vi "2-5.vi"() -> ()   [LabVIEW 2022 SP3]
panel:
  out "高压报警警示灯":bool
  out "正常运行指示灯":bool
  out "当前电压值":dbl
  out "当前电压报警上限值":dbl
  in  "确定按钮":bool
  in  "电压报警上限值":dbl
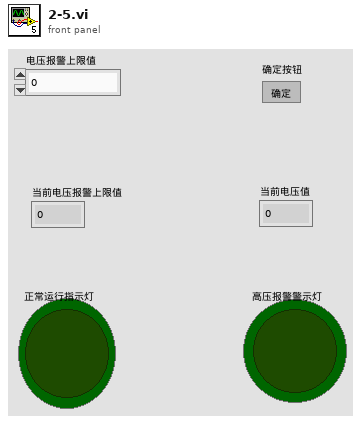
[diagram p1: front panel]
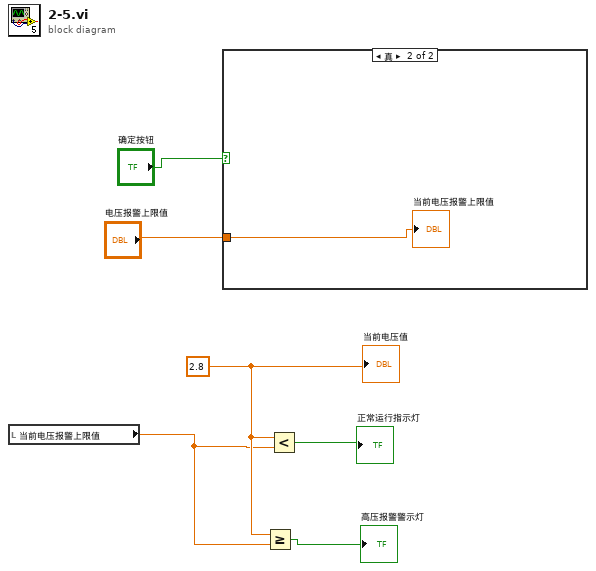
[diagram p0: block diagram]
diagram:
  w2 = 2.8
  n1 = local read "当前电压报警上限值"() -> (w1:dbl)
  n2 = case shown="真" "确定按钮" {
    tunnel: "电压报警上限值" -> [_ w7]
    frame False {
    }
    frame True {
      "当前电压报警上限值" <- w7
    }
  }
  n3 = Greater Or Equal?(x=w2, y=w1) -> (x >= y?=→"高压报警警示灯":bool)
  n4 = Less?(x=w2, y=w1) -> (x < y?=→"正常运行指示灯":bool)
  "当前电压值" <- w2
